vi "getTime.vi"(8 "error in (no error)":errorcluster) -> (0 "error out":errorcluster, 2 "timestamp":dbl, 3 "Monochromator out":refnum<class "Monochromator.lvclass">)   [LabVIEW 2016, in "Monochromator.lvclass"]
uses:
  Monochromator.lvclass
panel:
  in  "Monochromator in":refnum<class "Monochromator.lvclass">
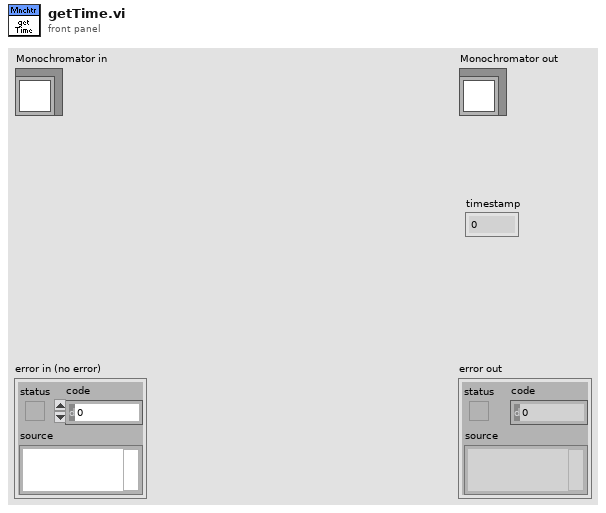
[diagram p1: front panel]
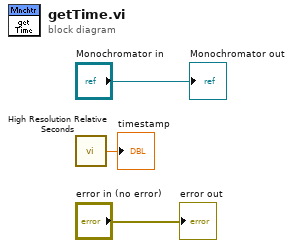
[diagram p0: block diagram]
diagram:
  n1 = call <vilib>:"High Resolution Relative Seconds.vi"() -> ("relative seconds"=→"timestamp":dbl)
  "error out" <- "error in (no error)"
  "Monochromator out" <- "Monochromator in"
